vi "Test Add Child UID To Parent List.vi"(8 "error in (no error)":errorcluster) -> (0 "error out":errorcluster)   [LabVIEW 2017, in "Unit Tests.lvlib"]
uses:
  Unit Tests.lvlib
  source/Browser Core/Server Classes/Base Tree/Base Tree.lvclass
  source/Browser Core/Node Classes/Generic Node/Generic Node.lvclass
  source/Browser Core/Server Classes/Base Tree/Base Tree.lvclass/Base Tree.ctl
  source/Browser Core/Node Classes/Generic Node/Generic Node.lvclass/Generic Node.ctl
  <vilib>/addons/_JKI Toolkits/Caraya/classes/Test/Test.lvclass
  <vilib>/addons/_JKI Toolkits/Caraya/classes/Assert/Assert.lvclass
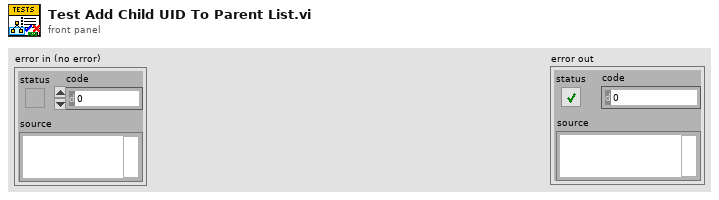
[diagram p1: front panel]
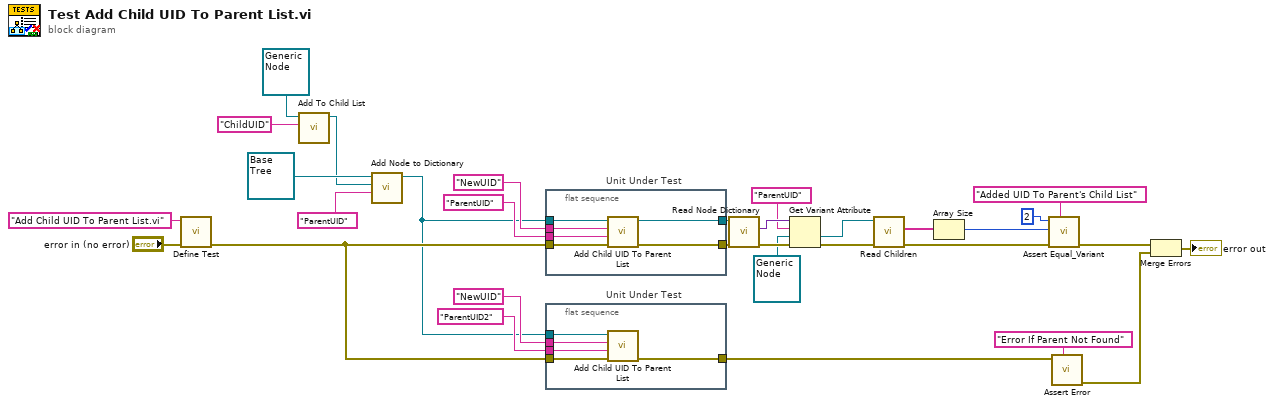
[diagram p0: block diagram]
diagram:
  n1 = call <vilib>:"Define Test.vi"("error in (no error)"="error in (no error)", "Label (VI Title)"="Add Child UID To Parent List.vi") -> ("error out"=w18:errorcluster)  [unwired: 9 in]
  n2 = call-dynamic "Add To Child List.vi"("Child ID"="ChildUID", "Generic Node in"=refnum<class "Generic Node.lvclass"> refnum ("New Node")) -> ("Generic Node out"=w10:refnum<class "Generic Node.lvclass">)  [unwired: 9 in]
  n3 = call "Add Node to Dictionary.vi"("UID"="ParentUID", "New Node"=w10, "Base Tree in"=refnum<class "Base Tree.lvclass"> refnum ("Browser Core.lvlib:Base Tree.lvclass")) -> ("Base Tree out"=w17:refnum<class "Base Tree.lvclass">)  [unwired: 8 in]
  n4 = flat-sequence "Unit Under Test" {
    tunnel: w18 -> [w37]
    tunnel: w17 -> [w36]
    tunnel: "ParentUID" -> [w35]
    tunnel: "NewUID" -> [w34]
    tunnel: [w33] -> w9
    tunnel: [w32] -> w8
    frame #0 {
      n5 = call "Add Child UID To Parent List.vi"("Base Tree in"=w36, "UID"=w34, "Parent"=w35, "error in (no error)"=w37) -> ("Base Tree out"=w32:refnum<class "Base Tree.lvclass">, "error out"=w33:errorcluster)  [unwired: 5 in]
    }
  }
  n6 = flat-sequence "Unit Under Test" {
    tunnel: w18 -> [w42]
    tunnel: w17 -> [w41]
    tunnel: "ParentUID2" -> [w40]
    tunnel: "NewUID" -> [w39]
    tunnel: [w38] -> w16
    frame #0 {
      n7 = call "Add Child UID To Parent List.vi"("Base Tree in"=w41, "UID"=w39, "Parent"=w40, "error in (no error)"=w42) -> ("error out"=w38:errorcluster)  [unwired: 5 in, 1 out]
    }
  }
  n8 = call "Read Node Dictionary.vi"("error in (no error)"=w9, "Base Tree in"=w8) -> ("error out"=w7:errorcluster, "Node Dictionary"=w6:variant)  [unwired: 7 in, 1 out]
  n9 = Get Variant Attribute(Variant=w6, name="ParentUID", default value (empty Variant)=refnum<class "Generic Node.lvclass"> refnum ("New Node"), error in=w7) -> (value=w2:refnum<class "Generic Node.lvclass">, error out=w4:errorcluster)  [unwired: 2 out]
  n10 = call "Read Children.vi"("error in (no error)"=w4, "Generic Node in"=w2) -> ("error out"=w14:errorcluster, "Children"=w15:string[])  [unwired: 7 in, 1 out]
  n11 = Array Size(array=w15) -> (size(s)=w12:i32)
  n12 = call <vilib>:"Assert Equal_Variant.vi"("Label"="Added UID To Parent's Child List", "error in (no error)"=w14, "Y"=w12, "X"=2 ("size(s)")) -> ("error out"=w13:errorcluster)  [unwired: 7 in]
  n13 = call <vilib>:"Assert Error.vi"("Label"="Error If Parent Not Found", "Error?"=w16) -> ("error out"=w30:errorcluster)  [unwired: 9 in]
  n14 = Merge Errors(w13, w30) -> (→"error out":errorcluster)
